vi "Panel Insert Subpanel.vi"(8 "error in (no error)":errorcluster, 10 "VI Refnum":refnum<vi>, 11 "Panel Control_Ref in":refnum<class "Panel Controller.lvclass">) -> (0 "error out":errorcluster, 3 "Panel Control_Ref out":refnum<class "Panel Controller.lvclass">)   [LabVIEW 2015, in "Panel Controller.lvclass"]
uses:
  Panel Controller.lvclass
panel:
  out "*(type *) &x":u16
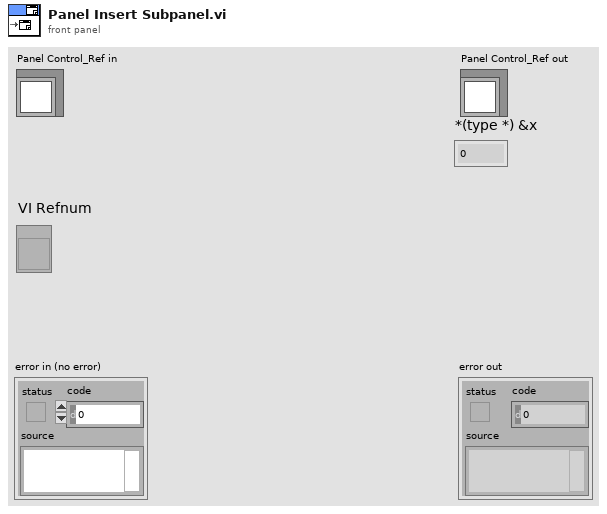
[diagram p1: front panel]
types:
  T1 = typedef "Panel Controller.lvclass/ObjectAttributes.ctl" = cluster{"Sub Panel Ref":refnum<vi>, "Panel_Q":refnum<queue>, "VI Running Refnum":refnum<vi>, "Brower Controller_Q":refnum<class "Message Enqueuer.lvclass">, "GUI Control Builder Director.lvclass":refnum<class "GUI Control Builder Director.lvclass">, "Panel GUI Manager.lvclass":refnum<class "Panel GUI Manager.lvclass">}
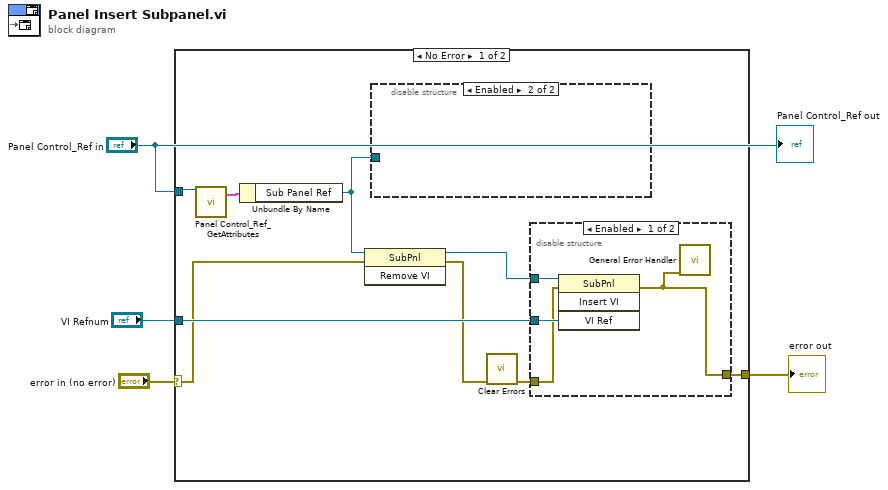
[diagram p0: block diagram]
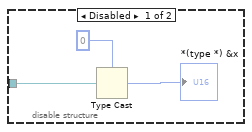
[diagram p2: hidden frame]
diagram:
  n1 = case shown="No Error" "error in (no error)" {
    selector: "error in (no error)" -> [w9 w21]
    tunnel: "VI Refnum" -> [w12 _]
    tunnel: [w11 w21] -> w2
    tunnel: "Panel Control_Ref in" -> [w10 _]
    frame No Error {
      n2 = call "Panel Control_Ref_GetAttributes.vi"("reference in"=w10) -> ("Data"=w13:T1)  [unwired: 15 in, 3 out]
      n3 = Unbundle By Name(w13) -> ("Sub Panel Ref"=w5:refnum<vi>)
      n4 = invoke class="SubPnl" method="Remove VI"(reference=w5, error in=w9) -> (reference out=w8:refnum<vi>, error out=w7:errorcluster)  [unwired: 1 in, 1 out]
      n5 = disable-structure shown="Enabled" {
        disable-tunnel: w5 -> [w16 _]
        frame Disabled {
          n6 = Type Cast(type=u16 0, x=w16) -> (*(type *) &x=→"*(type *) &x":u16)
        }
        frame Enabled {
        }
      }
      n7 = call <vilib>:"Clear Errors.vi"("error in (no error)"=w7) -> ("error out"=w6:errorcluster)  [unwired: 5 in, 1 out]
      n8 = disable-structure shown="Enabled" {
        disable-tunnel: w8 -> [w20 _]
        disable-tunnel: w12 -> [w19 _]
        disable-tunnel: w6 -> [w18 _]
        disable-tunnel: [w17 _] -> w11
        frame Enabled {
          n9 = invoke class="SubPnl" method="Insert VI"(reference=w20, error in=w18, "VI Ref"=w19) -> (error out=w17:errorcluster)  [unwired: 1 in, 3 out]
          n10 = call <vilib>:"General Error Handler.vi"("error in (no error)"=w17) -> ()  [unwired: 10 in, 5 out]
        }
        frame Disabled {
        }
      }
    }
    frame Error {
    }
  }
  "error out" <- w2
  "Panel Control_Ref out" <- "Panel Control_Ref in"
